vi "CIF proto Post-Install Custom Action.vi"(10 "Variant":variant) -> (0 "error out":errorcluster)   [LabVIEW 2021]
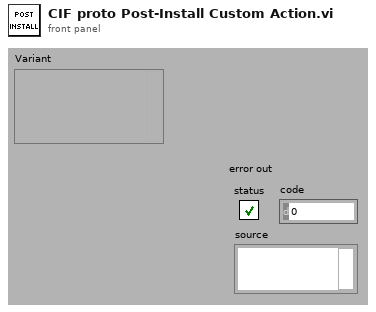
[diagram p1: front panel]
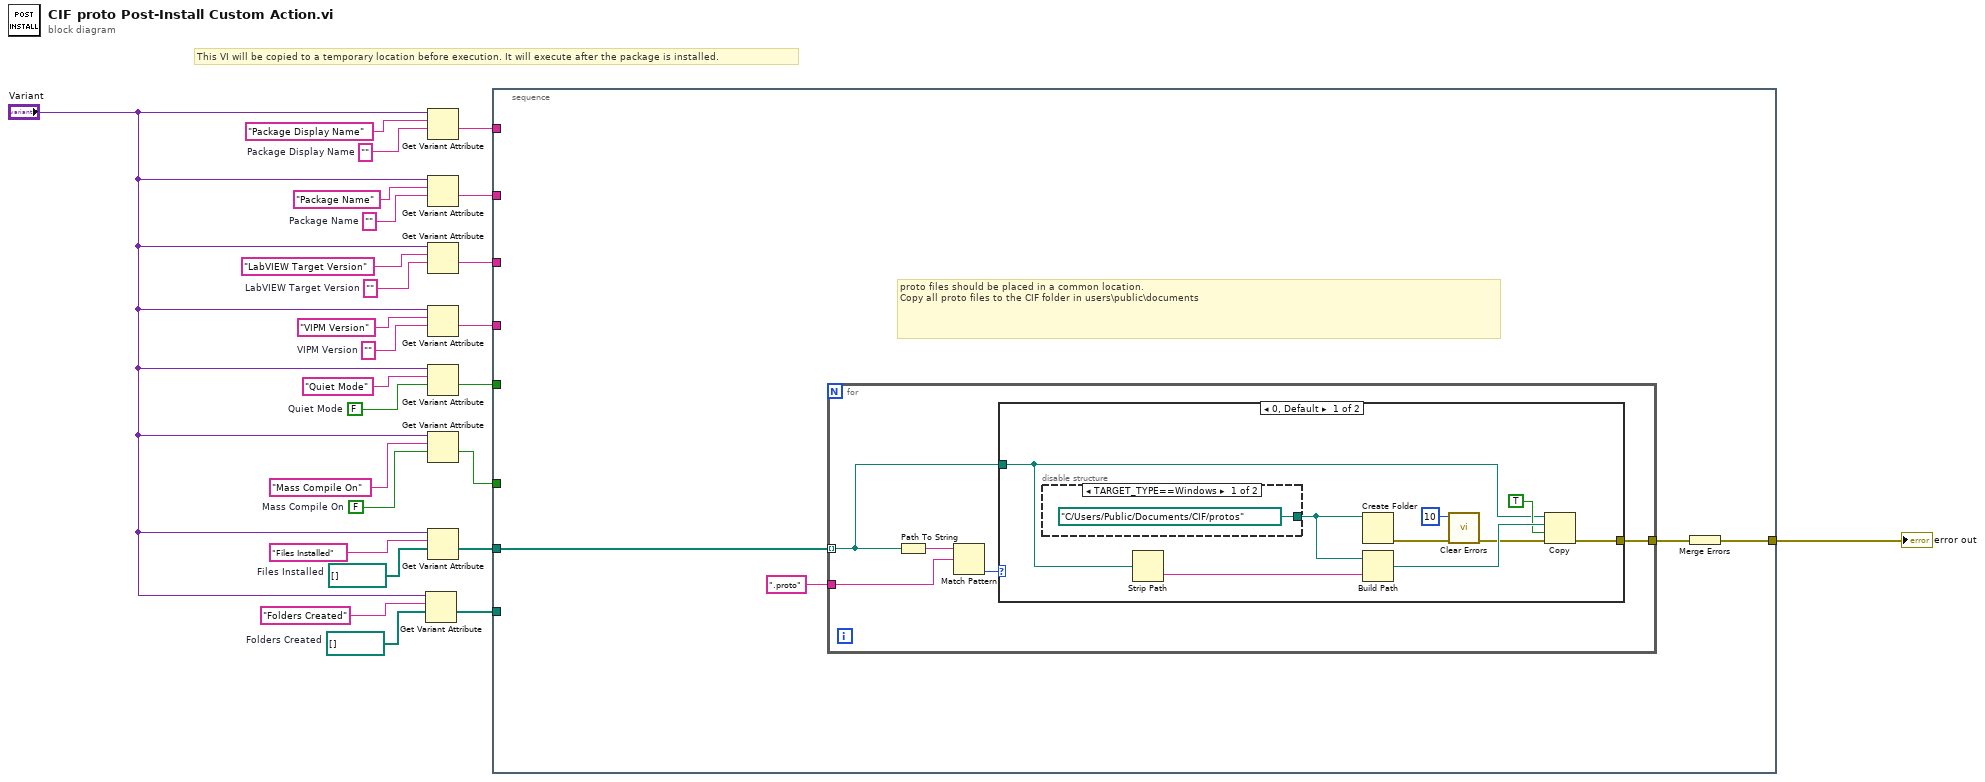
[diagram p0: block diagram]
diagram:
  w2 = path[] []  # Folders Created
  w3 = path[] []  # Files Installed
  w9 = FALSE  # Mass Compile On
  w10 = ""  # Package Display Name
  w17 = FALSE  # Quiet Mode
  w20 = ""  # VIPM Version
  w22 = ""  # LabVIEW Target Version
  w24 = ""  # Package Name
  # "This VI will be copied to a temporary location before execution. It will execute after the package is installed."
  n1 = Get Variant Attribute(Variant="Variant", name="Folders Created", default value (empty Variant)=w2) -> (value=w7:path[])  [unwired: 1 in, 3 out]
  n2 = Get Variant Attribute(Variant="Variant", name="Package Display Name", default value (empty Variant)=w10) -> (value=w16:string)  [unwired: 1 in, 3 out]
  n3 = Get Variant Attribute(Variant="Variant", name="Package Name", default value (empty Variant)=w24) -> (value=w15:string)  [unwired: 1 in, 3 out]
  n4 = Get Variant Attribute(Variant="Variant", name="LabVIEW Target Version", default value (empty Variant)=w22) -> (value=w14:string)  [unwired: 1 in, 3 out]
  n5 = Get Variant Attribute(Variant="Variant", name="VIPM Version", default value (empty Variant)=w20) -> (value=w13:string)  [unwired: 1 in, 3 out]
  n6 = Get Variant Attribute(Variant="Variant", name="Quiet Mode", default value (empty Variant)=w17) -> (value=w12:bool)  [unwired: 1 in, 3 out]
  n7 = Get Variant Attribute(Variant="Variant", name="Mass Compile On", default value (empty Variant)=w9) -> (value=w11:bool)  [unwired: 1 in, 3 out]
  n8 = Get Variant Attribute(Variant="Variant", name="Files Installed", default value (empty Variant)=w3) -> (value=w6:path[])  [unwired: 1 in, 3 out]
  n9 = stacked-sequence {
    tunnel: w16 -> [_]
    tunnel: w15 -> [_]
    tunnel: w14 -> [_]
    tunnel: w13 -> [_]
    tunnel: w12 -> [_]
    tunnel: w11 -> [_]
    tunnel: w6 -> [w30]
    tunnel: w7 -> [_]
    tunnel: [w28] -> w1
    frame #0 {
      # "proto files should be placed in a common location. \nCopy all proto files to the CIF folder in users\\public\\documents"
      n10 = for {
        tunnel: w30 -> [w31] mode=indexing
        tunnel: ".proto" ("regular expression") -> [w34]
        tunnel: [w32] -> w29
        n11 = Path To String(path=w31) -> (string=w35:string)
        n12 = Match Pattern(string=w35, regular expression=w34) -> (offset past match=w33:i32)  [unwired: 1 in, 3 out]
        n13 = case shown="0, Default" w33 {
          tunnel: w31 -> [w36 _]
          tunnel: [w42 _] -> w32
          frame 0, Default {
            n14 = disable-structure shown="TARGET_TYPE==Windows" {
              disable-tunnel: [path "C:/Users/Public/Documents/CIF/protos" ("configuration file path") _] -> w41
              frame condition #0 (active) {
              }
              frame condition #1 {
              }
            }
            n15 = Strip Path(path=w36) -> (name=w44:string)  [unwired: 1 out]
            n16 = Create Folder(path (use dialog)=w41) -> (error out=w40:errorcluster)  [unwired: 2 in, 2 out]
            n17 = Build Path(base path=w41, name or relative path=w44) -> (appended path=w43:path)
            n18 = call <vilib>:"Clear Errors.vi"("error in (no error)"=w40, "specific error code to clear (0: all)"=10) -> ("error out"=w39:errorcluster)  [unwired: 4 in, 1 out]
            n19 = Copy(8:w39, 9:TRUE ("overwrite (F)"), 10:w43, 11:w36) -> (0:w42:errorcluster)  [unwired: 1 in, 2 out]
          }
          frame -1 {
          }
        }
      }
      n20 = Merge Errors(w29) -> (w28:errorcluster)
    }
  }
  "error out" <- w1
